vi "MH_GetModuleInfo.vi"(8 "error in (no error)":errorcluster, 10 "modidx":i32, 11 "devidx":i32) -> (0 "error out":errorcluster, 1 "versioncode":i32, 2 "modelcode":i32, 3 "return type":i32)   [LabVIEW 2019]
uses:
  MH_DllPath_global.vi
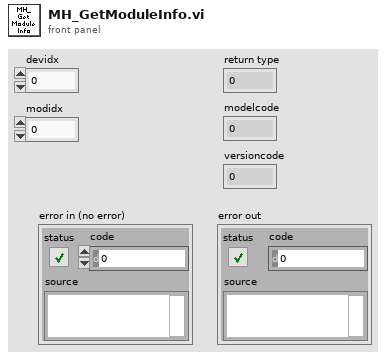
[diagram p1: front panel]
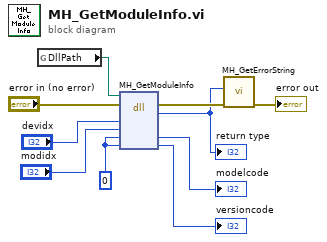
[diagram p0: block diagram]
diagram:
  w2 = 0 ("ctcstatus")
  n1 = global read "MH_DllPath_global.vi" "DllPath"() -> (w9:path)
  n2 = dll-call lib="MHLib64.dll" fn="MH_GetModuleInfo"(path in=w9, error in="error in (no error)", "devidx"="devidx", "modidx"="modidx", "modelcode"=w2, "versioncode"=w2) -> (error out=w7:errorcluster, "return type"=w6:i32, "modelcode"=→"modelcode":i32, "versioncode"=→"versioncode":i32)  [unwired: 3 in, 1 out]
  "return type" <- w6
  n3 = call "MH_GetErrorString.vi"("error in (no error)"=w7, "code"=w6) -> ("error out"=→"error out":errorcluster)  [unwired: 7 in, 2 out]
